vi "Find Gaps On Particular Machine.vi"(10 "Number of Scheduled Jobs on This Machine":i32, 11 "Gannt Chart For Machine In":T1[](array[typedef])) -> (3 "Gaps":T2[](array[typedef]))   [LabVIEW 2013, in "GA.lvclass"]
uses:
  GA.lvclass
  Controls/Gap.ctl
  Controls/GanntChart_Element.ctl
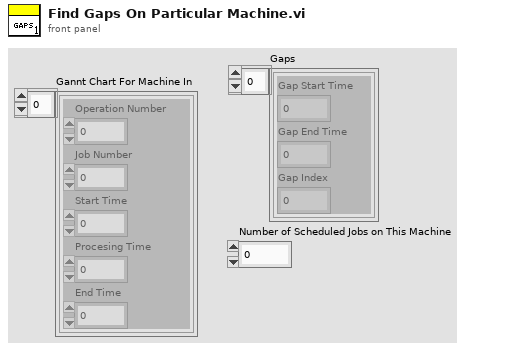
[diagram p1: front panel]
types:
  T1 = typedef "GanntChart_Element.ctl" = cluster{"Operation Number":i32, "Job Number":i32, "Start Time":i32, "Procesing Time":u16, "End Time":i32}
  T2 = typedef "Gap.ctl" = cluster{"Gap Start Time":i32, "Gap End Time":i32, "Gap Index":i32}
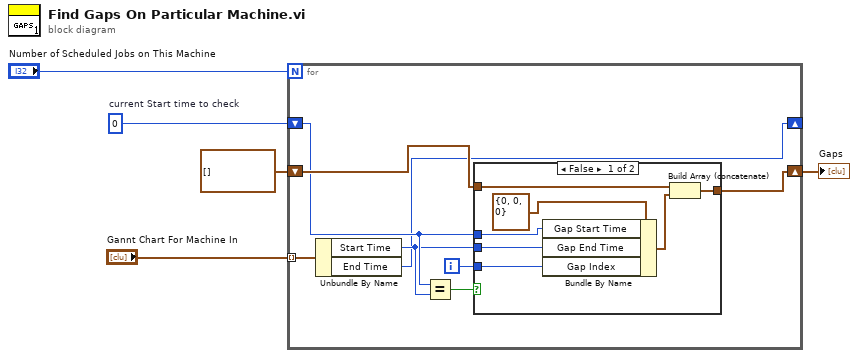
[diagram p0: block diagram]
diagram:
  w4 = 0  # current Start time to check
  n1 = for {
    N: "Number of Scheduled Jobs on This Machine" -> [_]
    tunnel: "Gannt Chart For Machine In" -> [w13] mode=indexing
    shift-right: [w7] -> _
    shift-left: w4 -> [w10]
    shift-right: [w8] -> w2
    shift-left: T2[] [] -> [w11]
    i -> [w6]
    n2 = Unbundle By Name(w13) -> ("Start Time"=w9:i32, "End Time"=w7:i32)
    n3 = Equal?(x=w10, y=w9) -> (x = y?=w12:bool)
    n4 = case shown="False" w12 {
      tunnel: w11 -> [w17 w21]
      tunnel: w10 -> [w19 _]
      tunnel: w9 -> [w18 _]
      tunnel: [w15 w21] -> w8
      tunnel: w6 -> [w14 _]
      frame False {
        n5 = Bundle By Name(cluster=T2 {"Gap Start Time"=0, "Gap End Time"=0, "Gap Index"=0}, "Gap Start Time"=w19, "Gap End Time"=w18, "Gap Index"=w14) -> (w16:T2)
        n6 = Build Array (concatenate)(w17, w16) -> (w15:T2[])
      }
      frame True {
      }
    }
  }
  "Gaps" <- w2
